vi "Laurel Modbus Read Rate Only.vi"(8 "error in (no error)":errorcluster, 11 "Modbus Master in":refnum<class "Modbus Master.lvclass">) -> (0 "error out":errorcluster, 2 "Rate":dbl, 3 "Modbus Master out":refnum<class "Modbus Master.lvclass">)   [LabVIEW 2020]
uses:
  <vilib>/NI/Modbus Library/API/Master/Modbus Master.lvclass
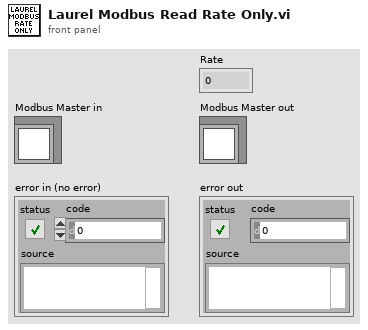
[diagram p1: front panel]
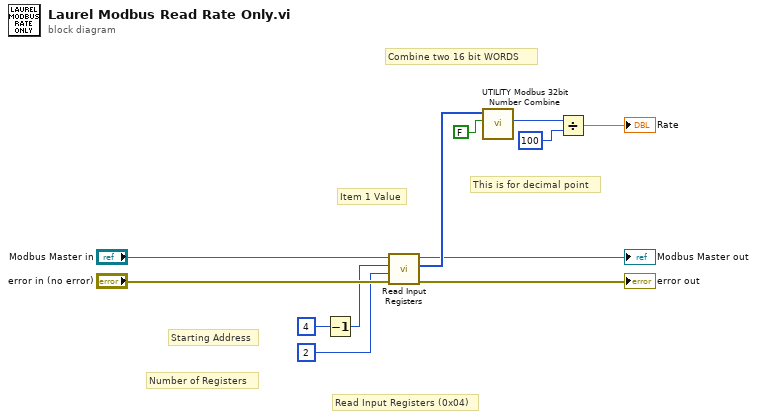
[diagram p0: block diagram]
diagram:
  # "This is for decimal point"
  # "Combine two 16 bit WORDS"
  # "Starting Address"
  # "Number of Registers"
  # "Read Input Registers (0x04)"
  # "Item 1 Value"
  n1 = Decrement(x=u16 4 ("starting address 2")) -> (x-1=w5:u16)
  n2 = call-dynamic "Read Input Registers.vi"("error in"="error in (no error)", "number of inputs"=u16 2, "starting address"=w5, "Modbus master in"="Modbus Master in") -> ("error out"=→"error out":errorcluster, "register values"=w7:u16[], "Modbus master out"=→"Modbus Master out":refnum<class "Modbus Master.lvclass">)  [unwired: 5 in]
  n3 = call "UTILITY Modbus 32bit Number Combine.vi"("Swap Words"=FALSE, "Holding Registers"=w7) -> ("word swapped"=w9:u32)  [unwired: 8 in, 1 out]
  n4 = Divide(x=w9, y=u32 100) -> (x/y=→"Rate":dbl)
